vi "generateTrapeze.vi"() -> (2 "Ramp Pattern":dbl[](graph))   [LabVIEW 2011]
uses:
  <vilib>/Analysis/1siggen.llb/Ramp Pattern by Samples.vi
  <vilib>/Analysis/NI_AALBase.lvlib
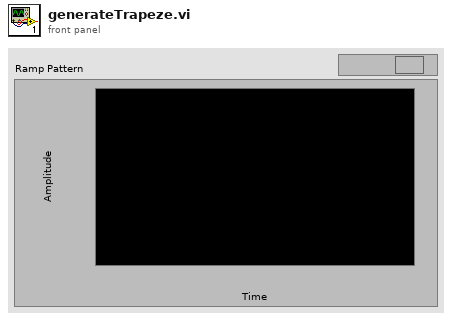
[diagram p1: front panel]
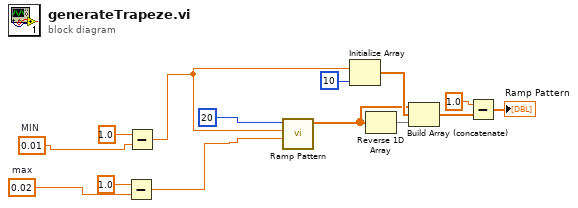
[diagram p0: block diagram]
diagram:
  w3 = 0.02  # max
  w5 = 0.01  # MIN
  n1 = Subtract(x=1.0, y=w3) -> (x-y=w2:dbl)
  n2 = Subtract(x=1.0, y=w5) -> (x-y=w1:dbl)
  n3 = call-poly <vilib>:"Ramp Pattern.vi"("start"=w2, "end"=w1, "samples"=20) -> ("Ramp Pattern"=w11:dbl[])  [unwired: 7 in, 1 out]
  n4 = Initialize Array(w1, 10 ("samples")) -> (w12:dbl[])
  n5 = Reverse 1D Array(array=w11) -> (reversed array=w10:dbl[])
  n6 = Build Array (concatenate)(w11, w12, w10) -> (w8:dbl[])
  n7 = Subtract(x=1.0, y=w8) -> (x-y=→"Ramp Pattern":dbl[])
